vi "Stop.vi"(6 "Teller":refnum<class "Teller.lvclass">, 8 "Error in":errorcluster, 9 "Parent Stopped":bool, 10 "Safe Stop":bool=TRUE, 11 "Core Actor in":refnum<class "Core Actor.lvclass">) -> (0 "Error out":errorcluster, 3 "Core Actor out":refnum<class "Core Actor.lvclass">)   [LabVIEW 2025, in "jettl.lvlib" / "Base Actor.lvlib" / "Core Actor.lvclass"]
uses:
  Core Actor.lvclass
  Teller/Teller.lvclass
  Core Actor.lvclass/Core Actor.ctl
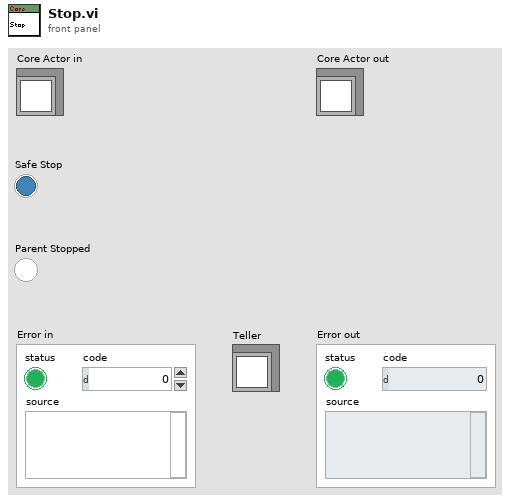
[diagram p1: front panel]
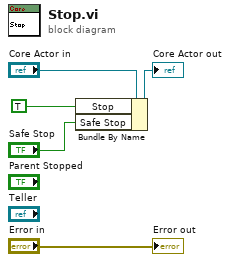
[diagram p0: block diagram]
diagram:
  n1 = Bundle By Name(cluster="Core Actor in", "Stop"=TRUE ("Is Marked For Destroy"), "Safe Stop"="Safe Stop") -> (→"Core Actor out":refnum<class "Core Actor.lvclass">)
  "Error out" <- "Error in"
